vi "fgv_erp42_serial.vi"(7 "cmd":enum16{"init", "read", "write", "close"}(ring), 8 "error in":errorcluster, 10 "count":i32) -> (0 "error out":errorcluster, 1 "ERP_Receive":T2, 2 "val":bool, 3 "read_buffer":string)   [LabVIEW 2019]
uses:
  Ctrl/erp42_receive_packet.ctl
  Ctrl/protocol_erp42.ctl
  <vilib>/Instr/_visa.llb/VISA Configure Serial Port (Instr).vi
panel:
  out "Drive_value":T1
  out "send_data":u8[](array[numeric]) format="%x"
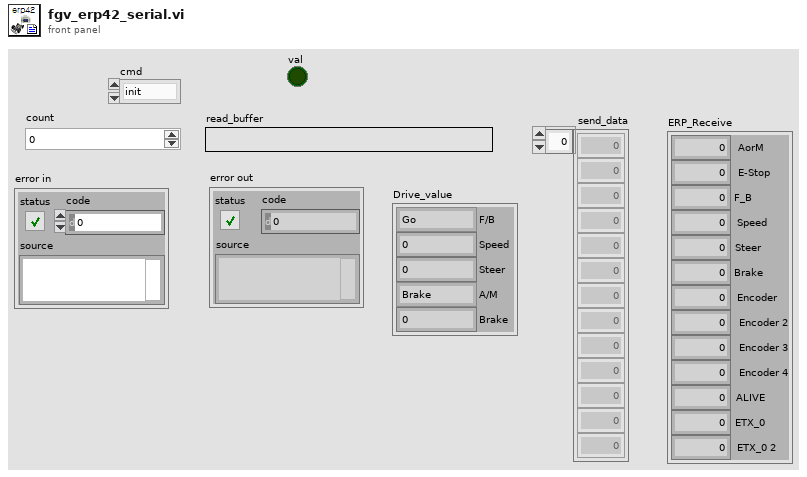
[diagram p1: front panel]
types:
  T1 = cluster{"F/B":enum16{"Go", "N", "Back"}, "Speed":u16, "Steer":i16, "A/M":enum16{"Brake", "Auto", "Manual"}, "Brake":u8}
  T2 = typedef "erp42_receive_packet.ctl" = cluster{"AorM":u8, "E-Stop":u8, "F_B":u8, "Speed":u16, "Steer":i16, "Brake":u8, "Encoder":u8, "Encoder 2":u8, "Encoder 3":u8, "Encoder 4":u8, "ALIVE":u8, "ETX_0":u8, "ETX_0 2":u8}
  T3 = typedef "protocol_erp42.ctl" = cluster{"S":u8, "T":u8, "X":u8, "AorM":u8, "E-Stop":u8, "F_B":u8, "Speed":u16, "Steer":i16, "Brake":u8, "ALIVE":u8, "ETX_0":u8, "ETX_0 2":u8}
  T4 = cluster{"Port":refnum<visa-resource-name>, "limits":cluster{"speed limits":cluster{"max":dbl, "min":dbl}, "steer limits":cluster{"width":dbl, "offset":dbl}}}
  T5 = typedef "data.ctl" = cluster{"Drive_value":cluster{"F/B":enum16{"Go", "N", "Back"}, "Speed":u16, "Steer":i16, "A/M":enum16{"Brake", "Auto", "Manual"}, "Brake":u8}}
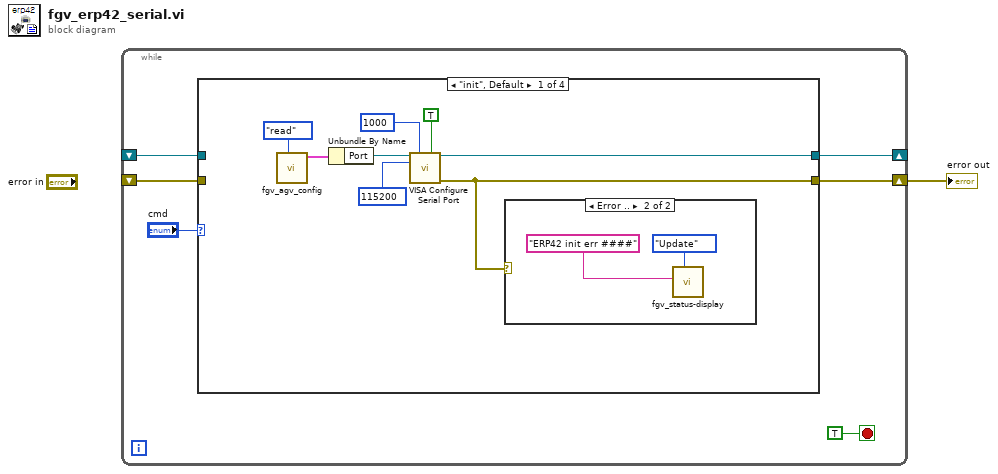
[diagram p0: block diagram]
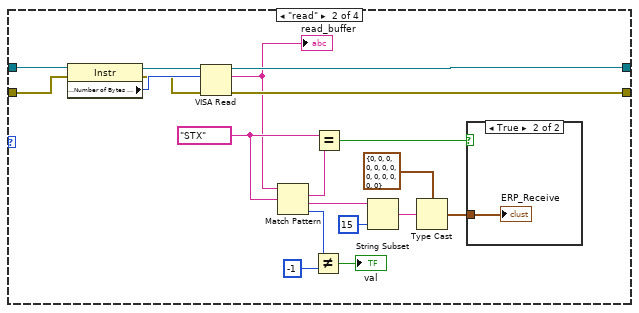
[diagram p3: hidden frame]
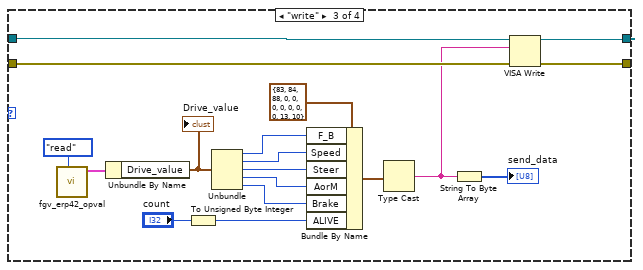
[diagram p5: hidden frame]
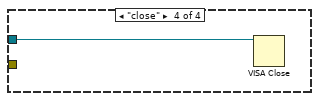
[diagram p6: hidden frame]
diagram:
  n1 = while {
    shift-right: [w5] -> _
    shift-left: _ -> [w3]
    shift-right: [w4] -> w1
    shift-left: _ -> [w2]
    stop <- TRUE stop-if-true
    n2 = case shown="\"init\", Default" "cmd" {
      tunnel: [w14 w33 w53 _] -> w5
      tunnel: [w8 w32 w52 _] -> w4
      tunnel: w3 -> [_ w36 w54 w56]
      tunnel: w2 -> [_ w30 w55 _]
      frame "init", Default {
        n3 = call "fgv_agv_config.vi"("cmd"=enum16{"read", "write"}."read") -> ("AGV cfg out"=w10:T4)  [unwired: 9 in, 1 out]
        n4 = Unbundle By Name(w10) -> ("Port"=w9:refnum<visa-resource-name>)
        n5 = call-poly "VISA Configure Serial Port"("VISA resource name"=w9, "timeout (10sec)"=u32 1000, "Enable Termination\nChar (T)"=TRUE ("Enable Termination\nChar (T)"), "baud rate (9600)"=u32 115200) -> ("VISA resource name out"=w14:refnum<visa-resource-name>, "error out"=w8:errorcluster)  [unwired: 10 in]
        n6 = case shown="Error .." w8 {
          frame No Error {
          }
          frame Error {
            n7 = call "fgv_status-display.vi"("Mode"=enum16{"Initial", "Update", "Clear"}."Update", "title"="ERP42 init err ####" ("String in")) -> ()  [unwired: 9 in, 1 out]
          }
        }
      }
      frame "read" {
        w24 = "STX" ("검색 문자열/문자 (-)")
        n8 = property class="Instr"(reference=w36, error in=w30) -> (reference out=w34:refnum<visa-resource-name>, error out=w31:errorcluster, "Serial Settings:Number of Bytes at Serial Port"=w35:u32)
        n9 = VISA Read(VISA resource name=w34, byte count=w35, error in (no error)=w31) -> (VISA resource name out=w33:refnum<visa-resource-name>, read buffer=w22:string, error out=w32:errorcluster)  [unwired: 1 out]
        "read_buffer" <- w22
        n10 = Match Pattern(string=w22, regular expression=w24) -> (match substring=w26:string, after substring=w25:string, offset past match=w20:i32)  [unwired: 1 in, 1 out]
        n11 = Not Equal?(x=w20, y=-1) -> (x != y?=→"val":bool)
        n12 = Equal?(x=w24, y=w26) -> (x = y?=w27:bool)
        n13 = String Subset(string=w25, length (rest)=15 ("길이(나머지)")) -> (substring=w28:string)  [unwired: 1 in]
        n14 = Type Cast(type=T2 {"AorM"=0, "E-Stop"=0, "F_B"=0, "Speed"=0, "Steer"=0, "Brake"=0, "Encoder"=0, "Encoder 2"=0, "Encoder 3"=0, "Encoder 4"=0, "ALIVE"=0, "ETX_0"=0, "ETX_0 2"=0} ("ERP_Receive 3"), x=w28) -> (*(type *) &x=w29:T2)
        n15 = case shown="True" w27 {
          tunnel: w29 -> [_ w37]
          frame False {
          }
          frame True {
            "ERP_Receive" <- w37
          }
        }
      }
      frame "write" {
        n16 = call "fgv_erp42_opval.vi"("cmd"=enum16{"read", "write", "ini"}."read") -> ("data_out"=w49:T5)  [unwired: 10 in]
        n17 = Unbundle By Name(w49) -> ("Drive_value"=w48:T1)
        "Drive_value" <- w48
        n18 = To Unsigned Byte Integer(number="count") -> (unsigned 8bit integer=w41:u8)
        n19 = Unbundle(w48) -> ("F/B"=w47:enum16{"Go", "N", "Back"}, "Speed"=w42:u16, "Steer"=w46:i16, "A/M"=w45:enum16{"Brake", "Auto", "Manual"}, "Brake"=w44:u8)
        n20 = Bundle By Name(cluster=T3 {"S"=83, "T"=84, "X"=88, "AorM"=0, "E-Stop"=0, "F_B"=0, "Speed"=0, "Steer"=0, "Brake"=0, "ALIVE"=0, "ETX_0"=13, "ETX_0 2"=10} ("Protocol"), "F_B"=w47, "Speed"=w42, "Steer"=w46, "AorM"=w45, "Brake"=w44, "ALIVE"=w41) -> (w43:T3)
        n21 = Type Cast(x=w43) -> (*(type *) &x=w39:string)  [unwired: 1 in]
        n22 = String To Byte Array(string=w39) -> (unsigned byte array=→"send_data":u8[])
        n23 = VISA Write(VISA resource name=w54, write buffer=w39, error in (no error)=w55) -> (VISA resource name out=w53:refnum<visa-resource-name>, error out=w52:errorcluster)  [unwired: 1 out]
      }
      frame "close" {
        n24 = VISA Close(VISA resource name=w56) -> ()  [unwired: 1 in, 1 out]
      }
    }
  }
  "error out" <- w1
